vi "Graph Enable Disable Y-Scale.vi"(8 "error in":errorcluster, 11 "Graph Ref in":refnum<vi>) -> (0 "error out":errorcluster, 3 "Graph Ref in":refnum<vi>)   [LabVIEW 2023]
doc: "Use this VI to enable or disable the Y-scales based on plot visibility."
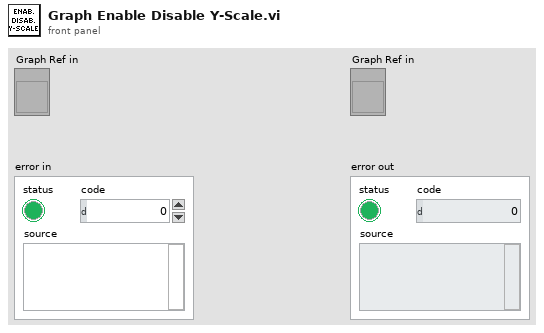
[diagram p1: front panel]
types:
  T1 = cluster{"Load currents":dbl[], "Efficiency":dbl[]}[]
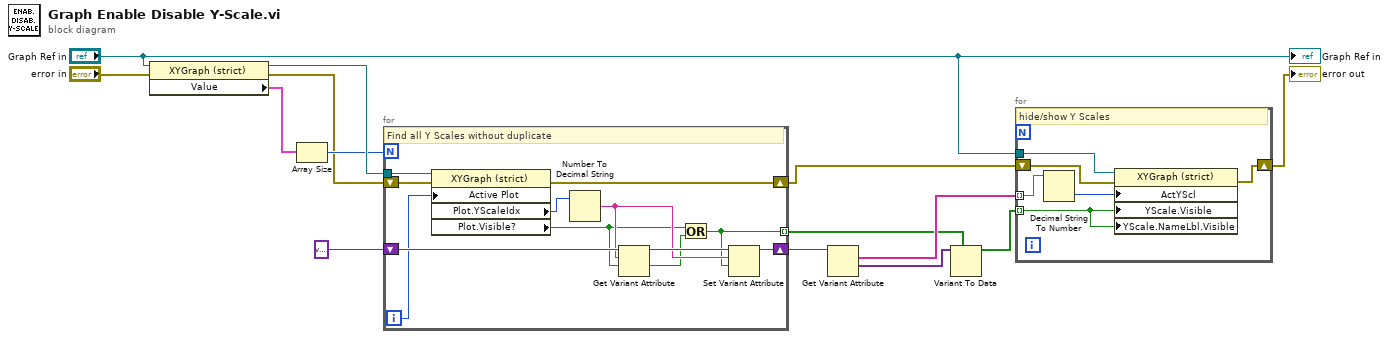
[diagram p0: block diagram]
diagram:
  n1 = property class="XYGraph (strict)"(reference="Graph Ref in", error in="error in") -> (reference out=w7:refnum<vi>, error out=w4:errorcluster, "Value"=w8:T1)
  n2 = Array Size(array=w8) -> (size(s)=w6:i32)
  n3 = for {
    N: w6 -> [_]
    shift-right: [w24] -> w13
    shift-left: variant ("variant") -> [w26]
    tunnel: [w22] -> w10 mode=indexing
    tunnel: w7 -> [w21]
    shift-right: [w15] -> w3
    shift-left: w4 -> [w16]
    i -> [w19]
    # "Find all Y Scales without duplicate"
    n4 = property class="XYGraph (strict)"(reference=w21, error in=w16, "Active Plot"=w19) -> (error out=w15:errorcluster, "Plot.YScaleIdx"=w20:u32, "Plot.Visible?"=w18:bool)  [unwired: 1 out]
    n5 = Number To Decimal String(number=w20) -> (decimal integer string=w23:string)  [unwired: 1 in]
    n6 = Get Variant Attribute(Variant=w26, name=w23, default value (empty Variant)=w18) -> (duplicate Variant=w25:variant, value=w17:bool)  [unwired: 1 in, 2 out]
    n7 = Or(x=w18, y=w17) -> (x .or. y?=w22:bool)
    n8 = Set Variant Attribute(Variant=w25, name=w23, value=w22) -> (Variant out=w24:variant)  [unwired: 1 in, 2 out]
  }
  n9 = Get Variant Attribute(Variant=w13) -> (names=w11:string[], values=w12:variant[])  [unwired: 3 in, 2 out]
  n10 = Variant To Data(type=w10, Variant=w12) -> (data=w9:bool[])  [unwired: 1 in, 1 out]
  n11 = for {
    tunnel: w11 -> [w32] mode=indexing
    tunnel: w9 -> [w27] mode=indexing
    tunnel: "Graph Ref in" -> [w31]
    shift-right: [w28] -> w2
    shift-left: w3 -> [w29]
    # "hide/show Y Scales"
    n12 = Decimal String To Number(string=w32) -> (number=w30:i32)  [unwired: 2 in, 1 out]
    n13 = property class="XYGraph (strict)"(reference=w31, error in=w29, "ActYScl"=w30, "YScale.Visible"=w27, "YScale.NameLbl.Visible"=w27) -> (error out=w28:errorcluster)  [unwired: 1 out]
  }
  "error out" <- w2
  "Graph Ref in" <- "Graph Ref in"
